vi "Set Speed and Acceleration.vi"(4 "Units (0: data)":u16(ring) items=["data", "microns/s, microns/s^2", "mm/s, mm/s^2", "inches/s, inches/s^2"], 5 "New Acceleration (0)":dbl, 7 "New Speed (0)":dbl, 8 "error in (no error)":errorcluster, 9 "Device and Axis":string, 10 "Microstep Size (0)":dbl, 11 "VISA resource name":refnum<visa-resource-name>) -> (0 "error out":errorcluster, 3 "VISA resource name out":refnum<visa-resource-name>)   [LabVIEW 2013, in "Zaber A Series.lvlib"]
doc: "Sets the speed and/or acceleration of a device to a new value. The desired speed and accel are inputs. If either is not connected or the value is 0, then it won't be updated. The units for the speed and acceleration can be selected with the Units input. 'Data' units are the default, and other unit selections require the Microstep Size for the device to be input. If you'd like to specify a Device and Axis to adjust the settings of, specify this input.\n\nThis VI requires that the Initialize VI has been called with the same serial port."
uses:
  Zaber A Series.lvlib
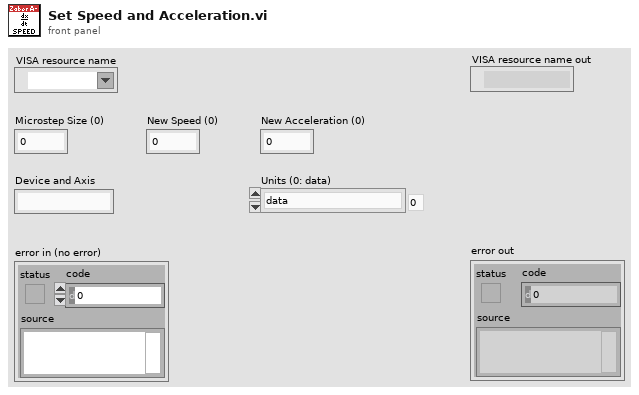
[diagram p1: front panel]
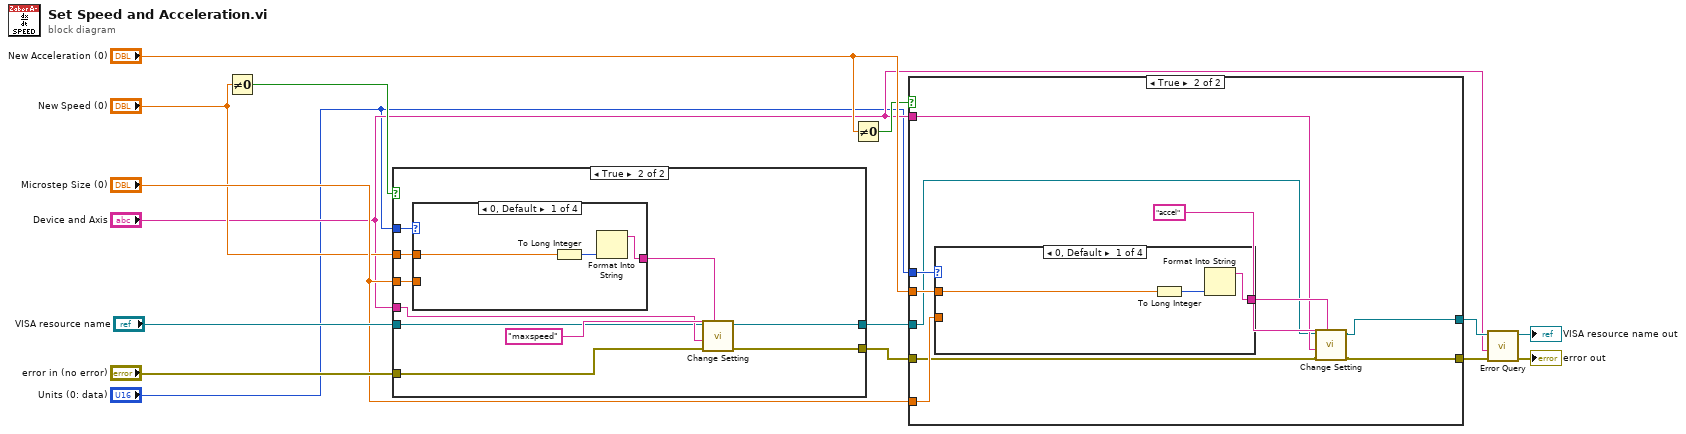
[diagram p0: block diagram]
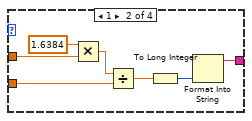
[diagram p3: hidden frame]
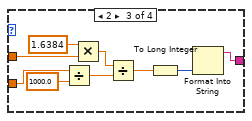
[diagram p4: hidden frame]
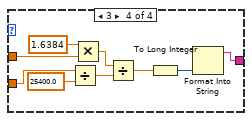
[diagram p5: hidden frame]
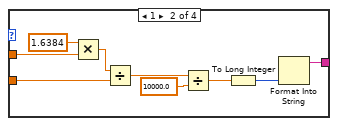
[diagram p7: hidden frame]
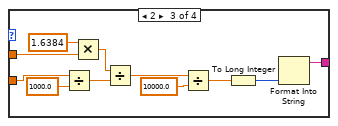
[diagram p8: hidden frame]
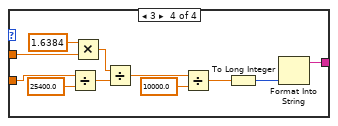
[diagram p9: hidden frame]
diagram:
  n1 = Not Equal To 0?(x="New Speed (0)") -> (x != 0?=w9:bool)
  n2 = case shown="True" w9 {
    tunnel: "VISA resource name" -> [w17 w20]
    tunnel: "error in (no error)" -> [w16 w22]
    tunnel: "New Speed (0)" -> [_ w27]
    tunnel: "Microstep Size (0)" -> [_ w26]
    tunnel: "Units (0: data)" -> [_ w25]
    tunnel: [w17 w19] -> w13
    tunnel: [w16 w18] -> w12
    tunnel: "Device and Axis" -> [_ w21]
    frame False {
    }
    frame True {
      n3 = case shown="0, Default" w25 {
        tunnel: w27 -> [w28 w33 w43 w51]
        tunnel: [w29 w36 w45 w54] -> w24
        tunnel: w26 -> [_ w32 w41 w48]
        frame 0, Default {
          n4 = To Long Integer(number=w28) -> (32bit integer=w30:i32)
          n5 = Format Into String(w30) -> (resulting string=w29:string)  [unwired: 3 in, 1 out]
        }
        frame 1 {
          n6 = Multiply(x=1.6384, y=w33) -> (x*y=w34:dbl)
          n7 = Divide(x=w34, y=w32) -> (x/y=w31:dbl)
          n8 = To Long Integer(number=w31) -> (32bit integer=w37:i32)
          n9 = Format Into String(w37) -> (resulting string=w36:string)  [unwired: 3 in, 1 out]
        }
        frame 2 {
          n10 = Divide(x=w41, y=1000.0) -> (x/y=w39:dbl)
          n11 = Multiply(x=1.6384, y=w43) -> (x*y=w38:dbl)
          n12 = Divide(x=w38, y=w39) -> (x/y=w44:dbl)
          n13 = To Long Integer(number=w44) -> (32bit integer=w46:i32)
          n14 = Format Into String(w46) -> (resulting string=w45:string)  [unwired: 3 in, 1 out]
        }
        frame 3 {
          n15 = Divide(x=w48, y=25400.0) -> (x/y=w47:dbl)
          n16 = Multiply(x=1.6384, y=w51) -> (x*y=w52:dbl)
          n17 = Divide(x=w52, y=w47) -> (x/y=w50:dbl)
          n18 = To Long Integer(number=w50) -> (32bit integer=w55:i32)
          n19 = Format Into String(w55) -> (resulting string=w54:string)  [unwired: 3 in, 1 out]
        }
      }
      n20 = call "Change Setting.vi"("Data"=w24, "error in (no error)"=w22, "Device and Axis"=w21, "Setting"="maxspeed" ("Common Settings"), "VISA resource name"=w20) -> ("error out"=w18:errorcluster, "VISA resource name out"=w19:refnum<visa-resource-name>)  [unwired: 5 in]
    }
  }
  n21 = Not Equal To 0?(x="New Acceleration (0)") -> (x != 0?=w7:bool)
  n22 = case shown="True" w7 {
    tunnel: w13 -> [w57 w58]
    tunnel: [w57 w64] -> w6
    tunnel: w12 -> [w56 w62]
    tunnel: [w56 w63] -> w4
    tunnel: "Microstep Size (0)" -> [_ w67]
    tunnel: "New Acceleration (0)" -> [_ w66]
    tunnel: "Units (0: data)" -> [_ w65]
    tunnel: "Device and Axis" -> [_ w59]
    frame False {
    }
    frame True {
      n23 = case shown="0, Default" w65 {
        tunnel: w66 -> [w68 w74 w81 w91]
        tunnel: [w69 w78 w89 w100] -> w61
        tunnel: w67 -> [_ w73 w80 w92]
        frame 0, Default {
          n24 = To Long Integer(number=w68) -> (32bit integer=w70:i32)
          n25 = Format Into String(w70) -> (resulting string=w69:string)  [unwired: 3 in, 1 out]
        }
        frame 1 {
          n26 = Multiply(x=1.6384, y=w74) -> (x*y=w75:dbl)
          n27 = Divide(x=w75, y=w73) -> (x/y=w72:dbl)
          n28 = Divide(x=w72, y=10000.0) -> (x/y=w71:dbl)
          n29 = To Long Integer(number=w71) -> (32bit integer=w79:i32)
          n30 = Format Into String(w79) -> (resulting string=w78:string)  [unwired: 3 in, 1 out]
        }
        frame 2 {
          n31 = Divide(x=w80, y=1000.0) -> (x/y=w86:dbl)
          n32 = Multiply(x=1.6384, y=w81) -> (x*y=w85:dbl)
          n33 = Divide(x=w85, y=w86) -> (x/y=w84:dbl)
          n34 = Divide(x=w84, y=10000.0) -> (x/y=w83:dbl)
          n35 = To Long Integer(number=w83) -> (32bit integer=w90:i32)
          n36 = Format Into String(w90) -> (resulting string=w89:string)  [unwired: 3 in, 1 out]
        }
        frame 3 {
          n37 = Divide(x=w92, y=25400.0) -> (x/y=w99:dbl)
          n38 = Multiply(x=1.6384, y=w91) -> (x*y=w97:dbl)
          n39 = Divide(x=w97, y=w99) -> (x/y=w94:dbl)
          n40 = Divide(x=w94, y=10000.0) -> (x/y=w93:dbl)
          n41 = To Long Integer(number=w93) -> (32bit integer=w101:i32)
          n42 = Format Into String(w101) -> (resulting string=w100:string)  [unwired: 3 in, 1 out]
        }
      }
      n43 = call "Change Setting.vi"("Data"=w61, "error in (no error)"=w62, "Device and Axis"=w59, "Setting"="accel" ("Common Settings"), "VISA resource name"=w58) -> ("error out"=w63:errorcluster, "VISA resource name out"=w64:refnum<visa-resource-name>)  [unwired: 5 in]
    }
  }
  n44 = call "Error Query.vi"("error in (no error)"=w4, "Device and Axis"="Device and Axis", "VISA resource name"=w6) -> ("error out"=→"error out":errorcluster, "VISA resource name out"=→"VISA resource name out":refnum<visa-resource-name>)  [unwired: 5 in, 2 out]
